vi "test results.vi"(8 "test pass":bool, 9 "step_type":T1, 10 "Numeric":i32, 11 "(description) used in test":string) -> (3 "test results":T2)   [LabVIEW 2020]
uses:
  controls/test results.ctl
  controls/step_type.ctl
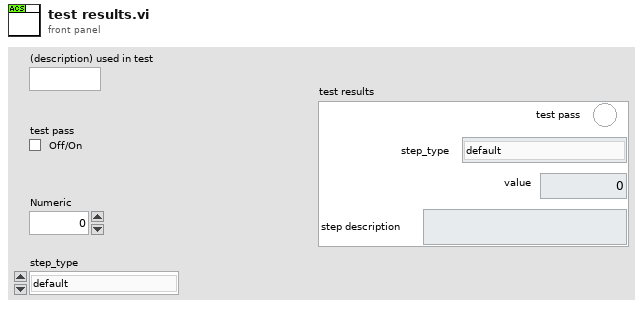
[diagram p1: front panel]
types:
  T1 = typedef "step_type.ctl" = enum16{"default", "prompt", "sequence#", "12V power supply on_off", "set_hipot_V", "set_hipot_I_limit", "set_hipot_ramping (sec)", "set hipot_hold_time", "read_hipot_V", "read_hipot_I", "set_daq", "read_daq", "flash uds", "wait (sec)", "record_pass_fail", "stop_test", "error_exit"}
  T2 = typedef "test results.ctl" = cluster{"test pass":bool, "step_type":T1, "value":dbl, "step description":string}
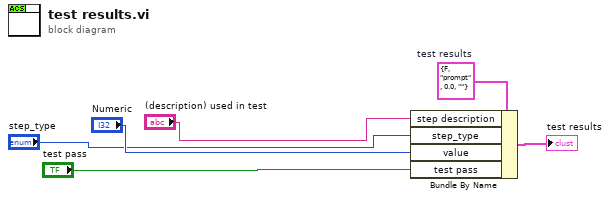
[diagram p0: block diagram]
diagram:
  w2 = T2 {"test pass"=FALSE, "step_type"=enum."prompt", "value"=0.0, "step description"=""}  # test results
  n1 = Bundle By Name(cluster=w2, "step description"="(description) used in test", "step_type"="step_type", "value"="Numeric", "test pass"="test pass") -> (→"test results":T2)
